vi "update stimulator config control (sub-vi).vi"(7 "odor config array":T1, 8 "error in (no error)":errorcluster, 9 "disable on error? (T)":bool=TRUE, 10 "re/initialize (F)":bool, 11 "manifold config array refnum":refnum<vi>) -> (0 "error out":errorcluster, 3 "manifold config array refnum out":refnum<vi>, 4 "value error out":errorcluster)   [LabVIEW 2021]
uses:
  type-defs/odor description array (type def).ctl
  type-defs/odor info cluster (type def).ctl
  type-defs/odor selection (type def).ctl
  type-defs/odor color (type def).ctl
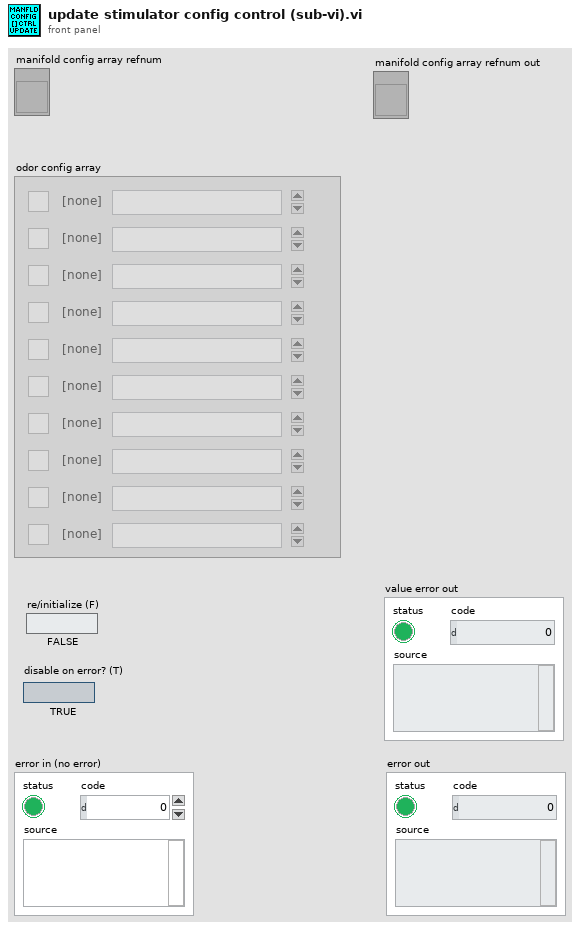
[diagram p1: front panel]
types:
  T1 = typedef "odor description array (type def).ctl" = T2[]
  T2 = typedef "odor info cluster (type def).ctl" = cluster{"odor channel":T3, "odor description":string, "odor color":T4, "odor channel active":bool}
  T3 = typedef "odor selection (type def).ctl" = enum16{"[none]", "odor 1", "odor 2", "odor 3", "odor 4", "odor 5", "odor 6", "odor 7", "odor 8", "odor 9", "odor 10"}
  T4 = typedef "odor color (type def).ctl" = u16
  T5 = enum8{"Enabled", "Disabled", "Disabled and Grayed Out"}
  T6 = typedef "odor channel to odor color map (type def).ctl" = map{T3, T4}
  T7 = typedef "stimulator configuration cluster (type def).ctl" = cluster{"position:":T8, "port connections:":T9[]}
  T8 = typedef "stimulator selection.ctl" = enum16{"left", "middle", "right"}
  T9 = typedef "single port single odor cluster.ctl" = cluster{"port number":T10, "connected odor":T3, "error":bool, "odor color":T4}
  T10 = typedef "port number (type def).ctl" = enum16{"port 1", "port 2", "port 3", "port 4", "port 5", "port 6", "port 7", "port 8"}
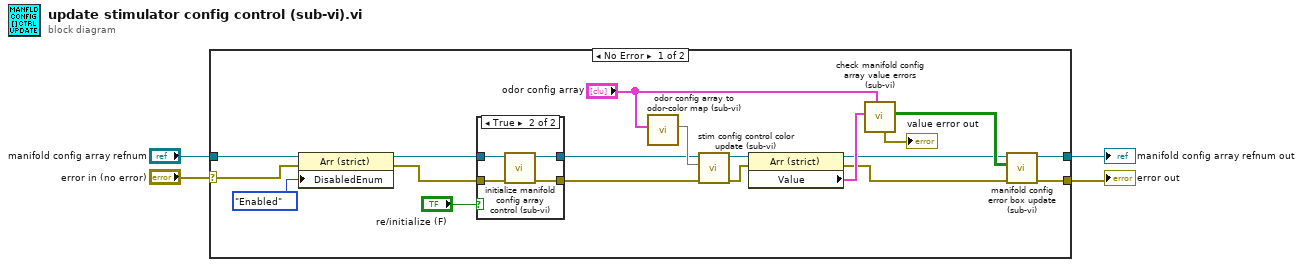
[diagram p0: block diagram]
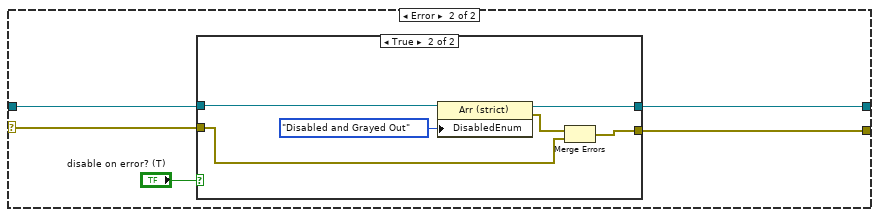
[diagram p3: hidden frame]
diagram:
  n1 = case shown="No Error" "error in (no error)" {
    selector: "error in (no error)" -> [w17 w30]
    tunnel: [w22 w31] -> w3
    tunnel: "manifold config array refnum" -> [w20 w33]
    tunnel: [w19 w32] -> w1
    frame No Error {
      n2 = property class="Arr (strict)"(reference=w20, error in=w17, "DisabledEnum"=T5."Enabled" ("Disabled")) -> (reference out=w16:refnum<vi>, error out=w15:errorcluster)
      n3 = case shown="True" "re/initialize (F)" {
        tunnel: w16 -> [w25 w29]
        tunnel: w15 -> [w24 w28]
        tunnel: [w25 w27] -> w14
        tunnel: [w24 w26] -> w13
        frame False {
        }
        frame True {
          n4 = call "initialize manifold config array control (sub-vi).vi"("error in (no error)"=w28, "stimulator config array refnum"=w29) -> ("error out"=w26:errorcluster, "stimulator config array refnum out"=w27:refnum<vi>)  [unwired: 8 in]
        }
      }
      n5 = call "odor config array to odor-color map (sub-vi).vi"("odor config array"="odor config array") -> ("odor-color map"=w21:T6)  [unwired: 10 in]
      n6 = call "stim config control color update (sub-vi).vi"("error in (no error)"=w13, "odor-color map"=w21, "maifold config array refnum"=w14) -> ("error out"=w9:errorcluster, "manifold config array refnum out"=w10:refnum<vi>)  [unwired: 7 in]
      n7 = property class="Arr (strict)"(reference=w10, error in=w9) -> (reference out=w6:refnum<vi>, error out=w5:errorcluster, "Value"=w7:T7[])
      n8 = call "check manifold config array value errors (sub-vi).vi"("odor config array"="odor config array", "manifold config array"=w7) -> ("manifold config error flag array"=w23:bool[][], "value error out"=→"value error out":errorcluster)  [unwired: 8 in]
      n9 = call "manifold config error box update (sub-vi).vi"("error in (no error)"=w5, "manifold config error array"=w23, "manifold config array refnum"=w6) -> ("error out"=w22:errorcluster, "manifold config array refnum out"=w19:refnum<vi>)  [unwired: 7 in]
    }
    frame Error {
      n10 = case shown="True" "disable on error? (T)" {
        tunnel: w33 -> [w36 w42]
        tunnel: [w36 w41] -> w32
        tunnel: [w35 w39] -> w31
        tunnel: w30 -> [w35 w38]
        frame False {
        }
        frame True {
          n11 = property class="Arr (strict)"(reference=w42, "DisabledEnum"=T5."Disabled and Grayed Out" ("Disabled")) -> (reference out=w41:refnum<vi>, error out=w40:errorcluster)  [unwired: 1 in]
          n12 = Merge Errors(w40, w38) -> (w39:errorcluster)
        }
      }
    }
  }
  "error out" <- w3
  "manifold config array refnum out" <- w1
